vi "ReadStepData.vi"(7 "error in (no error)":errorcluster, 10 "DataPath":path=path "C:/Users/Allen/Documents/Projects/NIST/Round Robin/FlukeResults/Excel/ILC 60_30 test results.xlsx") -> (0 "error out":errorcluster, 2 "PMUConfig":T1, 3 "Step Data":dbl[][][](array[numeric]) format="%#_9g")   [LabVIEW 2014]
uses:
  typedef/PMUConfig.ctl
  Excel(ActiveX)/enumOpenOrCreate.ctl
  Excel(ActiveX)/Excel(ActiveX).lvlib
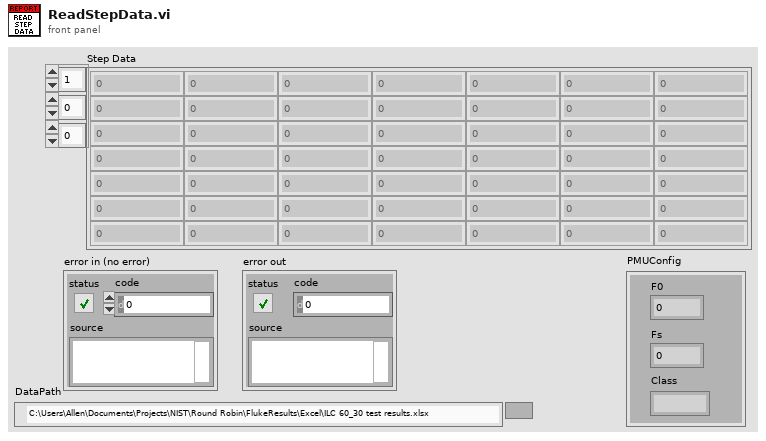
[diagram p1: front panel]
types:
  T1 = typedef "PMUConfig.ctl" = cluster{"Class":string, "Fs":dbl, "F0":dbl}
  T2 = typedef "Excel(ActiveX).lvlib/enumOpenOrCreate.ctl" = enum16{"open", "open or create", "create from template"}
  T3 = typedef "Excel(ActiveX).lvlib/ExcelActiveX.ctl" = cluster{"Excel._Application":refnum<k7>, "Application open at start":bool, "Excel._Worksheet":refnum<k7>, "Workbook open at start":bool, "Excel._Workbook":refnum<k7>, "Workbook Path":path, "Worksheet Name":string, "Row":u32, "Col":u32, "Cell":string, "Workbook Name":string}
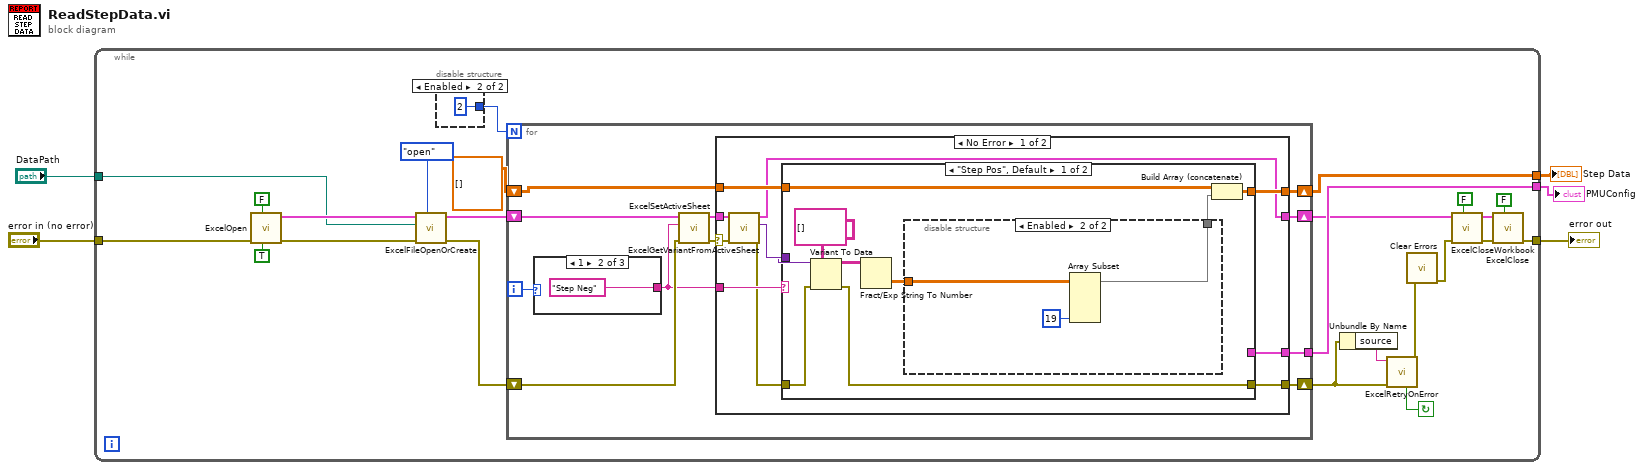
[diagram p0: block diagram]
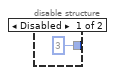
[diagram p2: hidden frame]
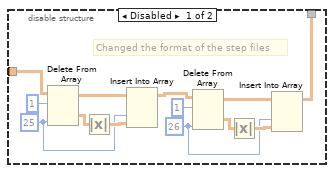
[diagram p3: hidden frame]
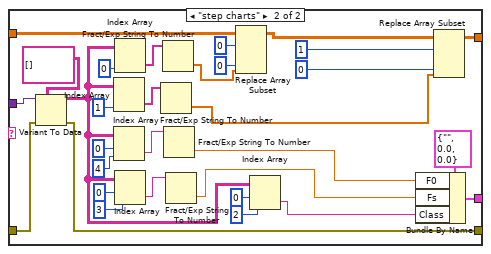
[diagram p4: hidden frame]
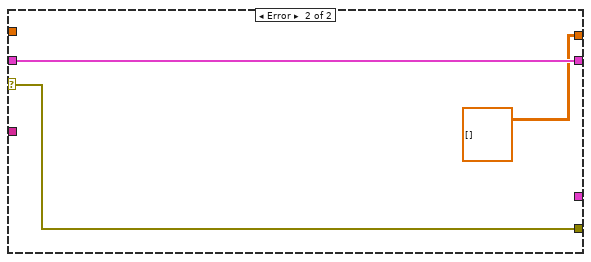
[diagram p5: hidden frame]
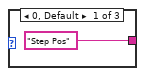
[diagram p6: hidden frame]
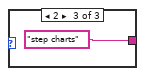
[diagram p7: hidden frame]
diagram:
  n1 = while {
    tunnel: "error in (no error)" -> [w28]
    tunnel: [w27] -> w4
    tunnel: [w16] -> w3
    tunnel: [w14] -> w2
    tunnel: "DataPath" -> [w7]
    stop <- w20 continue-if-true
    n2 = call "ExcelOpen.vi"("Run Minimized (f)"=TRUE ("Excel visible? (t)"), "Excel visible? (t)"=FALSE, "error in (no error)"=w28) -> ("error out"=w8:errorcluster, "ExcelActiveX"=w23:T3)  [unwired: 7 in]
    n3 = call "ExcelFileOpenOrCreate.vi"("Open or Create"=enumOpenOrCreate."open", "error in (no error)"=w8, "Excel file name and path"=w7, "ExcelActiveX in"=w23) -> ("error out"=w26:errorcluster, "ExcelActiveX out"=w25:T3)  [unwired: 6 in]
    n4 = disable-structure shown="Enabled" {
      disable-tunnel: [3 2] -> w6
      frame Disabled {
      }
      frame Enabled {
      }
    }
    n5 = for {
      N: w6 -> [_]
      shift-right: [w38] -> w11
      shift-left: w25 -> [w42]
      shift-right: [w37] -> w19
      shift-left: w26 -> [w41]
      shift-right: [w32] -> w16
      shift-left: dbl[][][] [] -> [w34]
      tunnel: [w33] -> w14
      i -> [w40]
      n6 = case shown="1" w40 {
        tunnel: ["Step Pos" "Step Neg" "step charts"] -> w35
        frame 0, Default {
        }
        frame 1 {
        }
        frame 2 {
        }
      }
      n7 = call "ExcelSetActiveSheet.vi"("error in (no error)"=w41, "Sheet Name"=w35, "ExcelActiveX in"=w42) -> ("error out"=w36:errorcluster, "ExcelActiveX  out"=w39:T3)  [unwired: 7 in]
      n8 = case shown="No Error" w36 {
        selector: w36 -> [w48 w110]
        tunnel: w39 -> [w47 w111]
        tunnel: [w46 w111] -> w38
        tunnel: [w52 w110] -> w37
        tunnel: w35 -> [w51 _]
        tunnel: [w50 dbl[][][] []] -> w32
        tunnel: w34 -> [w49 _]
        tunnel: [w45 _] -> w33
        frame No Error {
          n9 = call "ExcelGetVariantFromActiveSheet.vi"("error in (no error)"=w48, "ExcelActiveX  in"=w47) -> ("error out"=w43:errorcluster, "VariantOut"=w44:variant, "ExcelActiveX  out"=w46:T3)  [unwired: 7 in]
          n10 = case shown="\"Step Pos\", Default" w51 {
            tunnel: [w55 w90] -> w52
            tunnel: [w61 w79] -> w50
            tunnel: w49 -> [w60 w108]
            tunnel: w43 -> [w56 w91]
            tunnel: w44 -> [w58 w92]
            tunnel: [_ w93] -> w45
            frame "Step Pos", Default {
              n11 = Variant To Data(error in=w56, type=string[][] [], Variant=w58) -> (data=w57:string[][], error out=w55:errorcluster)
              n12 = Fract/Exp String To Number(string=w57) -> (number=w54:dbl[][])  [unwired: 3 in, 1 out]
              n13 = disable-structure shown="Enabled" {
                disable-tunnel: w54 -> [w74 w77]
                disable-tunnel: [w62 w76] -> w53
                frame Disabled {
                  w63 = 26 ("disabled index (col)")
                  w69 = 25 ("disabled index (col)")
                  # "Changed the format of the step files"
                  n14 = Delete From Array(array=w74, length=1, index (col)=w69) -> (deleted portion=w72:dbl[][], array with subset deleted=w71:dbl[][])  [unwired: 1 in]
                  n15 = Absolute Value(x=w72) -> (abs(x)=w70:dbl[][])
                  n16 = Insert Into Array(array=w71, index (col)=w69, new element=w70) -> (w64:dbl[][])  [unwired: 1 in]
                  n17 = Delete From Array(array=w64, length=1, index (col)=w63) -> (deleted portion=w66:dbl[][], array with subset deleted=w67:dbl[][])  [unwired: 1 in]
                  n18 = Absolute Value(x=w66) -> (abs(x)=w68:dbl[][])
                  n19 = Insert Into Array(array=w67, index (col)=w63, new element=w68) -> (w62:dbl[][])  [unwired: 1 in]
                }
                frame Enabled {
                  n20 = Array Subset(array=w77, length (col)=19 ("length")) -> (w76:dbl[][])  [unwired: 3 in]
                }
              }
              n21 = Build Array (concatenate)(w60, w53) -> (w61:dbl[][][])
            }
            frame "step charts" {
              n22 = Variant To Data(error in=w91, type=string[][] [], Variant=w92) -> (data=w89:string[][], error out=w90:errorcluster)
              n23 = Index Array(array=w89, index (col)=1 ("disabled index (col)")) -> (element=w85:string[])  [unwired: 1 in]
              n24 = Index Array(array=w89, index (row)=0, index (col)=4 ("disabled index (col)")) -> (element=w83:string)
              n25 = Index Array(array=w89, index (col)=0 ("disabled index (col)")) -> (element=w87:string[])  [unwired: 1 in]
              n26 = Index Array(array=w89, index (row)=0, index (col)=3 ("disabled index (col)")) -> (element=w81:string)
              n27 = Fract/Exp String To Number(string=w85) -> (number=w84:dbl[])  [unwired: 3 in, 1 out]
              n28 = Fract/Exp String To Number(string=w87) -> (number=w86:dbl[])  [unwired: 3 in, 1 out]
              n29 = Fract/Exp String To Number(string=w83) -> (number=w82:dbl)  [unwired: 3 in, 1 out]
              n30 = Fract/Exp String To Number(string=w81) -> (number=w80:dbl)  [unwired: 3 in, 1 out]
              n31 = Replace Array Subset(array=w108, new element=w86, index (dim 0)=0 ("index (page)"), index (dim 2)=0 ("disabled index (col)")) -> (w103:dbl[][][])  [unwired: 1 in]
              n32 = Index Array(array=w89, index (row)=0, index (col)=2 ("disabled index (col)")) -> (element=w78:string)
              n33 = Bundle By Name(cluster=T1 {"Class"="", "Fs"=0.0, "F0"=0.0} ("PMUConfig"), "F0"=w82, "Fs"=w80, "Class"=w78) -> (w93:T1)
              n34 = Replace Array Subset(array=w103, new element=w84, index (dim 0)=1 ("index (page)"), index (dim 2)=0 ("disabled index (col)")) -> (w79:dbl[][][])  [unwired: 1 in]
            }
          }
        }
        frame Error {
        }
      }
    }
    n35 = Unbundle By Name(w19) -> ("source"=w18:string)
    n36 = call "ExcelRetryOnError.vi"("error in (no error)"=w19, "Error Msg"=w18) -> ("error out"=w17:errorcluster, "Retry"=w20:bool)  [unwired: 8 in]
    n37 = call <vilib>:"Clear Errors.vi"("error in (no error)"=w17) -> ("error out"=w13:errorcluster)  [unwired: 5 in, 1 out]
    n38 = call "ExcelCloseWorkbook.vi"("Save"=FALSE, "error in (no error)"=w13, "ExcelActiveX"=w11) -> ("error out"=w12:errorcluster, "ExcelActiveX"=w10:T3)  [unwired: 7 in]
    n39 = call "ExcelClose.vi"("Leave Open (f)"=FALSE, "error in (no error)"=w12, "ExcelActiveX in"=w10) -> ("error out"=w27:errorcluster)  [unwired: 7 in, 1 out]
  }
  "error out" <- w4
  "Step Data" <- w3
  "PMUConfig" <- w2
